vi "NextPage.vi"(8 "error in (no error)":errorcluster, 11 "DataBase in":refnum<class "DataBase.lvclass">) -> (0 "error out":errorcluster, 3 "DataBase out":refnum<class "DataBase.lvclass">)   [LabVIEW 2019, in "DataBase.lvlib" / "DataBase.lvclass"]
uses:
  DataBase.lvclass
  DataBase.lvclass/DataBase.ctl
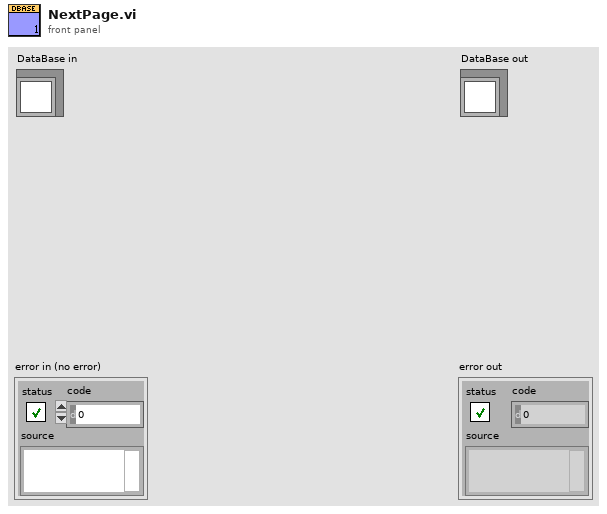
[diagram p1: front panel]
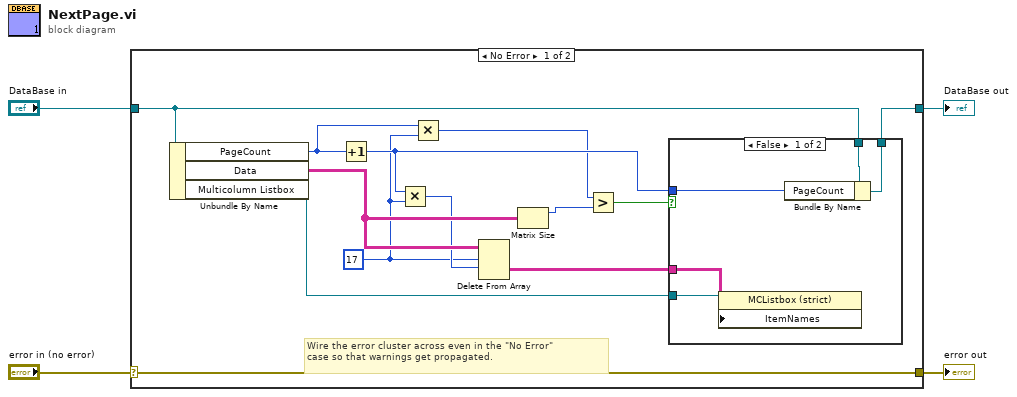
[diagram p0: block diagram]
diagram:
  n1 = case shown="No Error" "error in (no error)" {
    selector: "error in (no error)" -> [w17 w25]
    tunnel: [w17 w25] -> w3
    tunnel: [w8 w24] -> w1
    tunnel: "DataBase in" -> [w10 w24]
    frame No Error {
      w6 = 17 ("length")
      # "Wire the error cluster across even in the \"No Error\"\ncase so that warnings get propagated."
      n2 = Unbundle By Name(w10) -> ("PageCount"=w7:i32, "Data"=w14:string[][], "Multicolumn Listbox"=w16:refnum<vi>)
      n3 = Increment(x=w7) -> (x+1=w9:i32)
      n4 = Multiply(x=w9, y=w6) -> (x*y=w13:i32)
      n5 = Multiply(x=w7, y=w6) -> (x*y=w5:i32)
      n6 = Delete From Array(array=w14, length=w6, index (row)=w13) -> (deleted portion=w15:string[][])  [unwired: 1 in, 1 out]
      n7 = Matrix Size(0:w14) -> (1:w12:i32)  [unwired: 1 out]
      n8 = Greater?(x=w5, y=w12) -> (0:w11:bool)
      n9 = case shown="False" w11 {
        tunnel: w16 -> [w22 _]
        tunnel: w15 -> [w21 _]
        tunnel: w10 -> [w20 w23]
        tunnel: w9 -> [w19 _]
        tunnel: [w18 w23] -> w8
        frame False {
          n10 = property class="MCListbox (strict)"(reference=w22, "ItemNames"=w21) -> ()  [unwired: 1 in, 2 out]
          n11 = Bundle By Name(cluster=w20, "PageCount"=w19) -> (w18:refnum<class "DataBase.lvclass">)
        }
        frame True {
        }
      }
    }
    frame Error {
    }
  }
  "error out" <- w3
  "DataBase out" <- w1
